vi "Content_AddContent.vi"(8 "error in":errorcluster, 10 "Content":refnum<k24>, 11 "ContentCollection":refnum<k24>) -> (0 "error out":errorcluster, 3 "ContentCollection dup":refnum<k24>)   [LabVIEW 2009]
uses:
  C:/Projets/LAVAG/OpenOfficeRGT/AODL/DLLs/AODL.dll
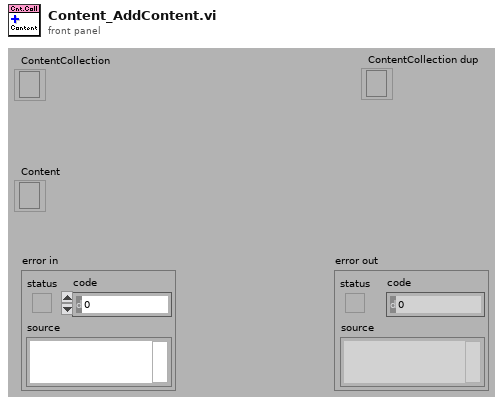
[diagram p1: front panel]
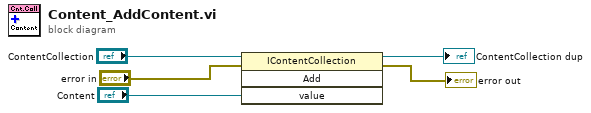
[diagram p0: block diagram]
diagram:
  n1 = invoke class="IContentCollection" method="Add"(reference="ContentCollection", error in="error in", "value"="Content") -> (reference out=→"ContentCollection dup":refnum<k24>, error out=→"error out":errorcluster)  [unwired: 1 in, 2 out]
